vi "Mission Time.vi"() -> (0 "MissionTime":dbl(knob) scale=0.0..10.0)   [LabVIEW 2010]
uses:
  5.0-Global.vi
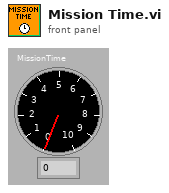
[diagram p1: front panel]
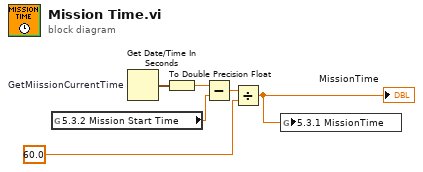
[diagram p0: block diagram]
diagram:
  n1 = global read "5.0-Global.vi" "5.3.2 Mission Start Time"() -> (w2:dbl)
  n2 = Get Date/Time In Seconds "GetMiissionCurrentTime"() -> (seconds since 1Jan1904=w4:timestamp)
  n3 = To Double Precision Float(number=w4) -> (double precision float=w5:dbl)
  n4 = Subtract(x=w5, y=w2) -> (x-y=w6:dbl)
  n5 = Divide(x=w6, y=60.0) -> (x/y=w3:dbl)
  "MissionTime" <- w3
  n6 = global write "5.0-Global.vi" "5.3.1 MissionTime"(w3) -> ()
